vi "GotoWaypoint.vi"(3 "SupressIn":dbl, 7 "InhibitIn":bool, 8 "CurrentSteerAngle":dbl, 9 "WhatAroundMe? Clean":cluster{"T":dbl, "Range":dbl, "Bearing":dbl}[](array[cluster]), 10 "WhereAmI? Clean":T2, 11 "MDF In":T1(array[cluster])) -> (0 "SupressOut":dbl, 1 "MDF Out":T1(array[cluster]), 2 "ActCommand":dbl[](array[numeric]), 4 "InhibitOut":bool, 5 "Vel":dbl, 6 "SteerAngle":dbl)   [LabVIEW 2010]
doc: "This subVI contains the Forebrain Goto Waypoint behaviors. Its inputs are the outputs of thewhat and where SENSE processes, theMission efinition Filet, a suppression value from another co-brahvior and an inhibit signal to turn the behavior off. The outputs are a 90 element steering array and a suppression value to diminish the output of co-behaviors.\n\nIt is designed to work with a 90 element behavior arbiter."
uses:
  <vilib>/Analysis/1siggen.llb/Ramp Pattern by Samples.vi
  <vilib>/gmath/statdist.llb/Normal PDF.vi
  <vilib>/gmath/NI_Gmath.lvlib
  <vilib>/Analysis/NI_AALBase.lvlib
panel:
  out "loop index":i32
  in  "HowAmI? Clean":cluster{"T":dbl, "Battery":dbl, "Temp":dbl}
  # "This VI contains the go to waypoint behavior  at the Forebrain level"
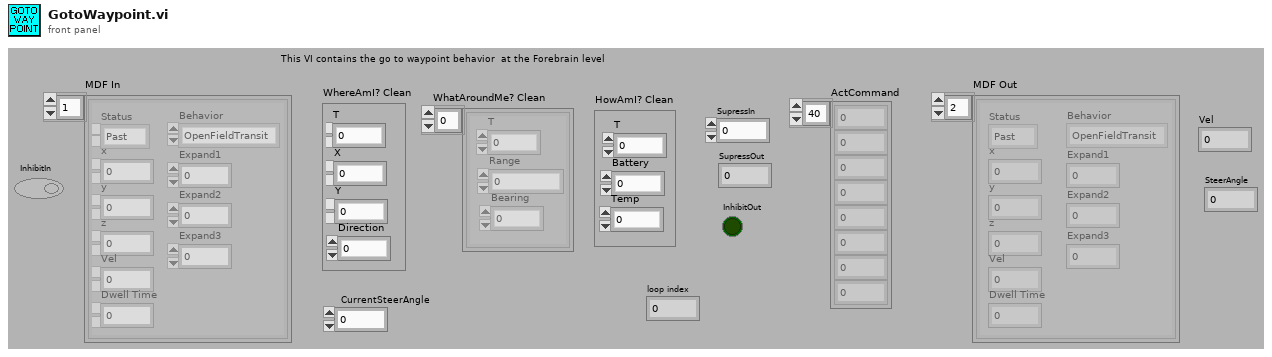
[diagram p1: front panel]
types:
  T1 = cluster{"Status":enum16{"Past", "Current", "Future"}, "x":dbl, "y":dbl, "z":dbl, "Vel":dbl, "Dwell Time":dbl, "Behavior":enum16{"OpenFieldTransit", "WallFollow", "LaneFollow", "ManualMode"}, "Expand1":dbl, "Expand2":dbl, "Expand3":dbl}[]
  T2 = cluster{"T":dbl, "X":dbl, "Y":dbl, "Direction":dbl}
  T3 = cluster{"VelCom":dbl, "BehCom":enum16{"OpenFieldTransit", "WallFollow", "LaneFollow", "ManualMode"}}
  T4 = cluster{"Status":enum16{"Past", "Current", "Future"}, "x":dbl, "y":dbl, "z":dbl, "Vel":dbl, "Dwell Time":dbl, "Behavior":enum16{"OpenFieldTransit", "WallFollow", "LaneFollow", "ManualMode"}, "Expand1":dbl, "Expand2":dbl, "Expand3":dbl}
  T5 = enum16{"OpenFieldTransit", "WallFollow", "LaneFollow", "ManualMode"}
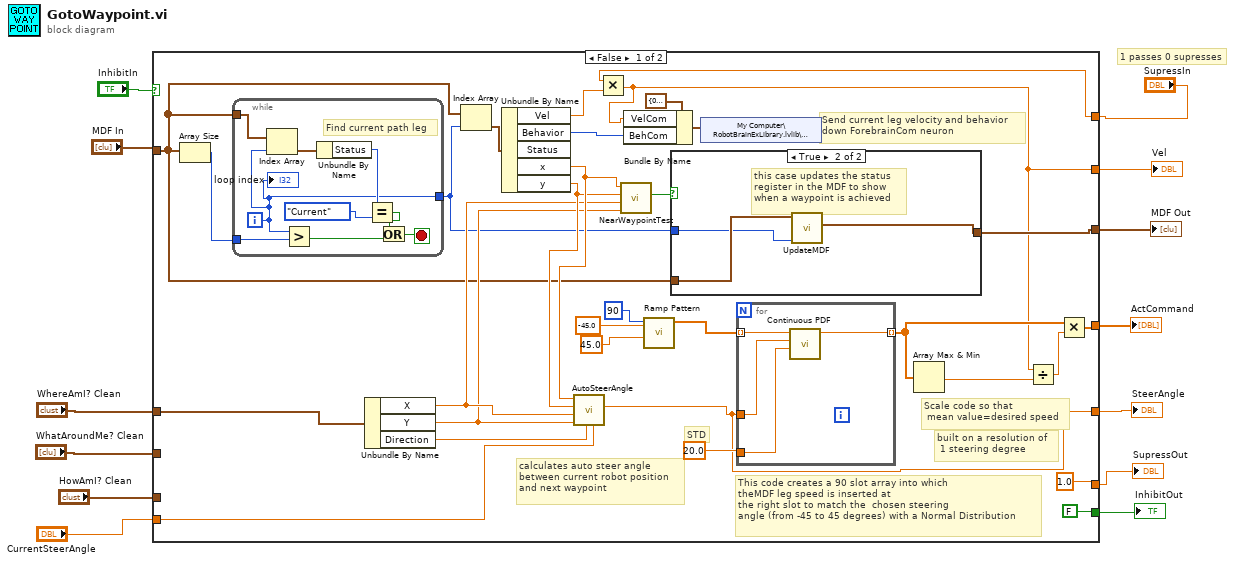
[diagram p0: block diagram]
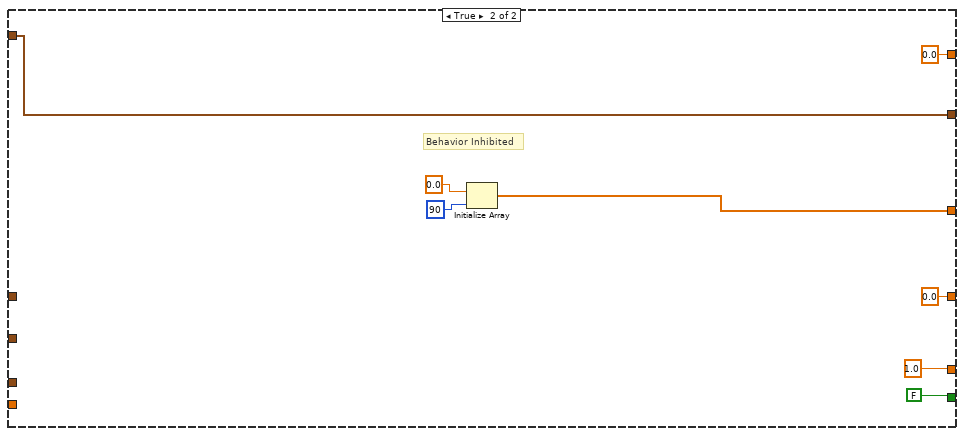
[diagram p3: hidden frame]
diagram:
  # "1 passes 0 supresses"
  n1 = case shown="False" "InhibitIn" {
    tunnel: "WhatAroundMe? Clean" -> [_ _]
    tunnel: "WhereAmI? Clean" -> [w41 _]
    tunnel: "HowAmI? Clean" -> [_ _]
    tunnel: "SupressIn" -> [w15 _]
    tunnel: [w28 w67] -> w6
    tunnel: [1.0 ("SupressOut") 1.0 ("SupressOut")] -> w8
    tunnel: [FALSE ("InhibitOut") FALSE ("InhibitOut")] -> w7
    tunnel: "MDF In" -> [w21 w64]
    tunnel: [w20 w64] -> w4
    tunnel: [w14 0.0 ("Vel")] -> w3
    tunnel: [w17 0.0 ("SteerAngle")] -> w2
    tunnel: "CurrentSteerAngle" -> [w16 _]
    frame False {
      # "calculates auto steer angle\nbetween current robot position\nand next waypoint"
      # "built on a resolution of\n 1 steering degree"
      # "Scale code so that\n mean value=desired speed"
      # "STD"
      # "This code creates a 90 slot array into which\ntheMDF leg speed is inserted at\nthe right slot to match the  chosen steering\nangle (from -45 to 45 degrees) with a Normal Distribution"
      # "Send current leg velocity and behavior\ndown ForebrainCom neuron"
      n2 = Array Size(array=w21) -> (size(s)=w42:i32)
      n3 = while {
        tunnel: w42 -> [w61]
        tunnel: w21 -> [w58]
        tunnel: [w53] -> w19
        i -> [w53]
        stop <- w60 stop-if-true
        # "Find current path leg"
        n4 = Index Array "Index Array"(array=w58, index=w53) -> (element=w55:T4)
        n5 = Greater?(x=w53, y=w61) -> (0:w59:bool)
        n6 = Unbundle By Name(w55) -> ("Status"=w56:enum16{"Past", "Current", "Future"})
        n7 = Equal?(x=w56, y=enum16{"Past", "Current", "Future"}."Current") -> (x = y?=w57:bool)
        n8 = Or(x=w57, y=w59) -> (x .or. y?=w60:bool)
        "loop index" <- w53
      }
      n9 = Unbundle By Name(w41) -> ("X"=w24:dbl, "Y"=w23:dbl, "Direction"=w27:dbl)
      n10 = Index Array "Index Array"(array=w21, index=w19) -> (element=w40:T4)
      n11 = Unbundle By Name(w40) -> ("Vel"=w18:dbl, "Behavior"=w37:T5, "x"=w26:dbl, "y"=w25:dbl)  [unwired: 1 out]
      n12 = call "AutoSteerAngle.vi"("CurrentSteerAngle"=w16, "CurrentDirection"=w27, "Ycurrent"=w23, "Xcurrent"=w24, "Ywaypoint"=w25, "Xwaypoint"=w26) -> ("NewSteerAngle"=w17:dbl)  [unwired: 5 in]
      n13 = Multiply(x=w15, y=w18) -> (x*y=w14:dbl)
      n14 = call "NearWaypointTest.vi"("Yrobot"=w23, "Xrobot"=w24, "Ywaypoint"=w25, "Xwaypoiny"=w26) -> ("AtWaypoint"=w22:bool)  [unwired: 7 in]
      n15 = Bundle By Name(cluster=T3 {"VelCom"=0.0, "BehCom"=enum."OpenFieldTransit"} ("ForebrainCom"), "VelCom"=w14, "BehCom"=w37) -> (w39:T3)
      n16 = call-poly <vilib>:"Ramp Pattern.vi"("start"=45.0, "end"=-45.0 ("end (Normal)"), "samples"=90) -> ("Ramp Pattern"=w31:dbl[])  [unwired: 7 in, 1 out]
      n17 = case shown="True" w22 {
        tunnel: w21 -> [w45 w48]
        tunnel: [w45 w46] -> w20
        tunnel: w19 -> [_ w47]
        frame False {
          # "robot not near waypoint\npass MDF through unaltered"
        }
        frame True {
          # "this case updates the status\nregister in the MDF to show \nwhen a waypoint is achieved"
          n18 = call "UpdateMDF.vi"("Index"=w47, "MDF_In"=w48) -> ("MDF_Out"=w46:T1)  [unwired: 9 in]
        }
      }
      n19 = shared-variable "My Computer\\RobotBrainExLibrary.lvlib\\ForebrainCom"(w39) -> ()  [unwired: 1 in, 1 out]
      n20 = for {
        tunnel: w31 -> [w52] mode=indexing
        tunnel: 20.0 ("std (Normal)") -> [w51]
        tunnel: [w50] -> w35 mode=indexing
        tunnel: w17 -> [w49]
        n21 = call-poly <vilib>:"Continuous PDF.vi"("std"=w51, "mean"=w49, "x"=w52) -> ("pdf(x)"=w50:dbl)  [unwired: 7 in, 1 out]
      }
      n22 = Array Max & Min(array=w35) -> (max value=w33:dbl)  [unwired: 3 out]
      n23 = Divide(x=w14, y=w33) -> (x/y=w34:dbl)
      n24 = Multiply(x=w35, y=w34) -> (x*y=w28:dbl[])
    }
    frame True {
      # "Behavior Inhibited"
      n25 = Initialize Array "Initialize Array"(0.0 ("element"), 90 ("dimension size")) -> (w67:dbl[])
    }
  }
  "ActCommand" <- w6
  "SupressOut" <- w8
  "InhibitOut" <- w7
  "MDF Out" <- w4
  "Vel" <- w3
  "SteerAngle" <- w2
